vi "Process_Comp_Data.vi"(6 "Queues":T14, 7 "One Seconds in":T11 {"Slave"."Ch1 High" format="%0.0f"; "Master"."Ch1 High" format="%0.0f"}, 8 "Status/Errors in":refnum<vi>, 9 "Get all messages?":bool=TRUE, 10 "Process data parameters out":T1={"Stop loop"={"Settings changed?"=FALSE, "Stop?"=refnum}, "Button refs"={"Stop program"=refnum, "Save settings"=refnum, "DAQ mode"=refnum, "Reset settings"=refnum, "Apply settings"=refnum, "Reset MAS"=refnum, "Reset SLV"=refnum, "Local DBase?"=refnum, "Last value DBase"=FALSE, "Database"=refnum, "Calibration"=refnum, "Save settings 2"=refnum}, "Process messages"={"Process message mode"=enum."Error", "Slave data?"=FALSE, "Length get settings message"=0, "Delta time"=0.0, "Data_Filter"={"Filter_Data"=FALSE, "Use_Thresh"=FALSE, "Reduce data?"=FALSE}, "Time_difference_stack"=[], "Starting sec"=0, "Ending sec"=0, "Ending sec 2"=0, "MAS_Page_Thresh"=refnum, "SLV_Page_Thresh"=refnum, "Database"=refnum}, "Settings state"={"MAS locked?"=refnum, "SLV locked?"=refnum}, "Mode"={"Mode"=enum."Dialog", "Expert?"=FALSE, "Dialog?"=FALSE}, "Alignment parameters"=refnum, "Timer parameters"=refnum, "Files"={"Path config file"=path "", "Path def. ini file"=path "", "Path ini file 1"=path "", "Path ini file 2"=path "", "Path RBF file"=path ""}, "Time difference"=refnum, "Alignment"={"GEN_Page_Calibrate"=refnum, "MAS_Page_Gain"=refnum, "MAS_Page_Offset"=refnum, "SLV_Page_Gain"=refnum, "SLV_Page_Offset"=refnum, "MAS_Page_Common"=refnum, "SLV_Page_Common"=refnum}, "Page Statistics"=refnum}, 11 "Devices in":T10) -> (0 "Status/Errors out":refnum<vi>, 3 "Devices out":T10)   [LabVIEW 2010]
uses:
  Controls/Devices.ctl
  Controls/Queues.ctl
  Controls/One_Second.ctl
  Controls/GPS_Timestamp.ctl
  Controls/One_Seconds.ctl
  Controls/Process_Data_Parameters.ctl
  Controls/Stop_Loop.ctl
  Controls/Button_Refs.ctl
  Controls/Process_Messages.ctl
  Controls/Process_Message_Mode.ctl
  Controls/Settings_State.ctl
  Controls/Mode.ctl
  Controls/Files.ctl
  Controls/Page_Calibration.ctl
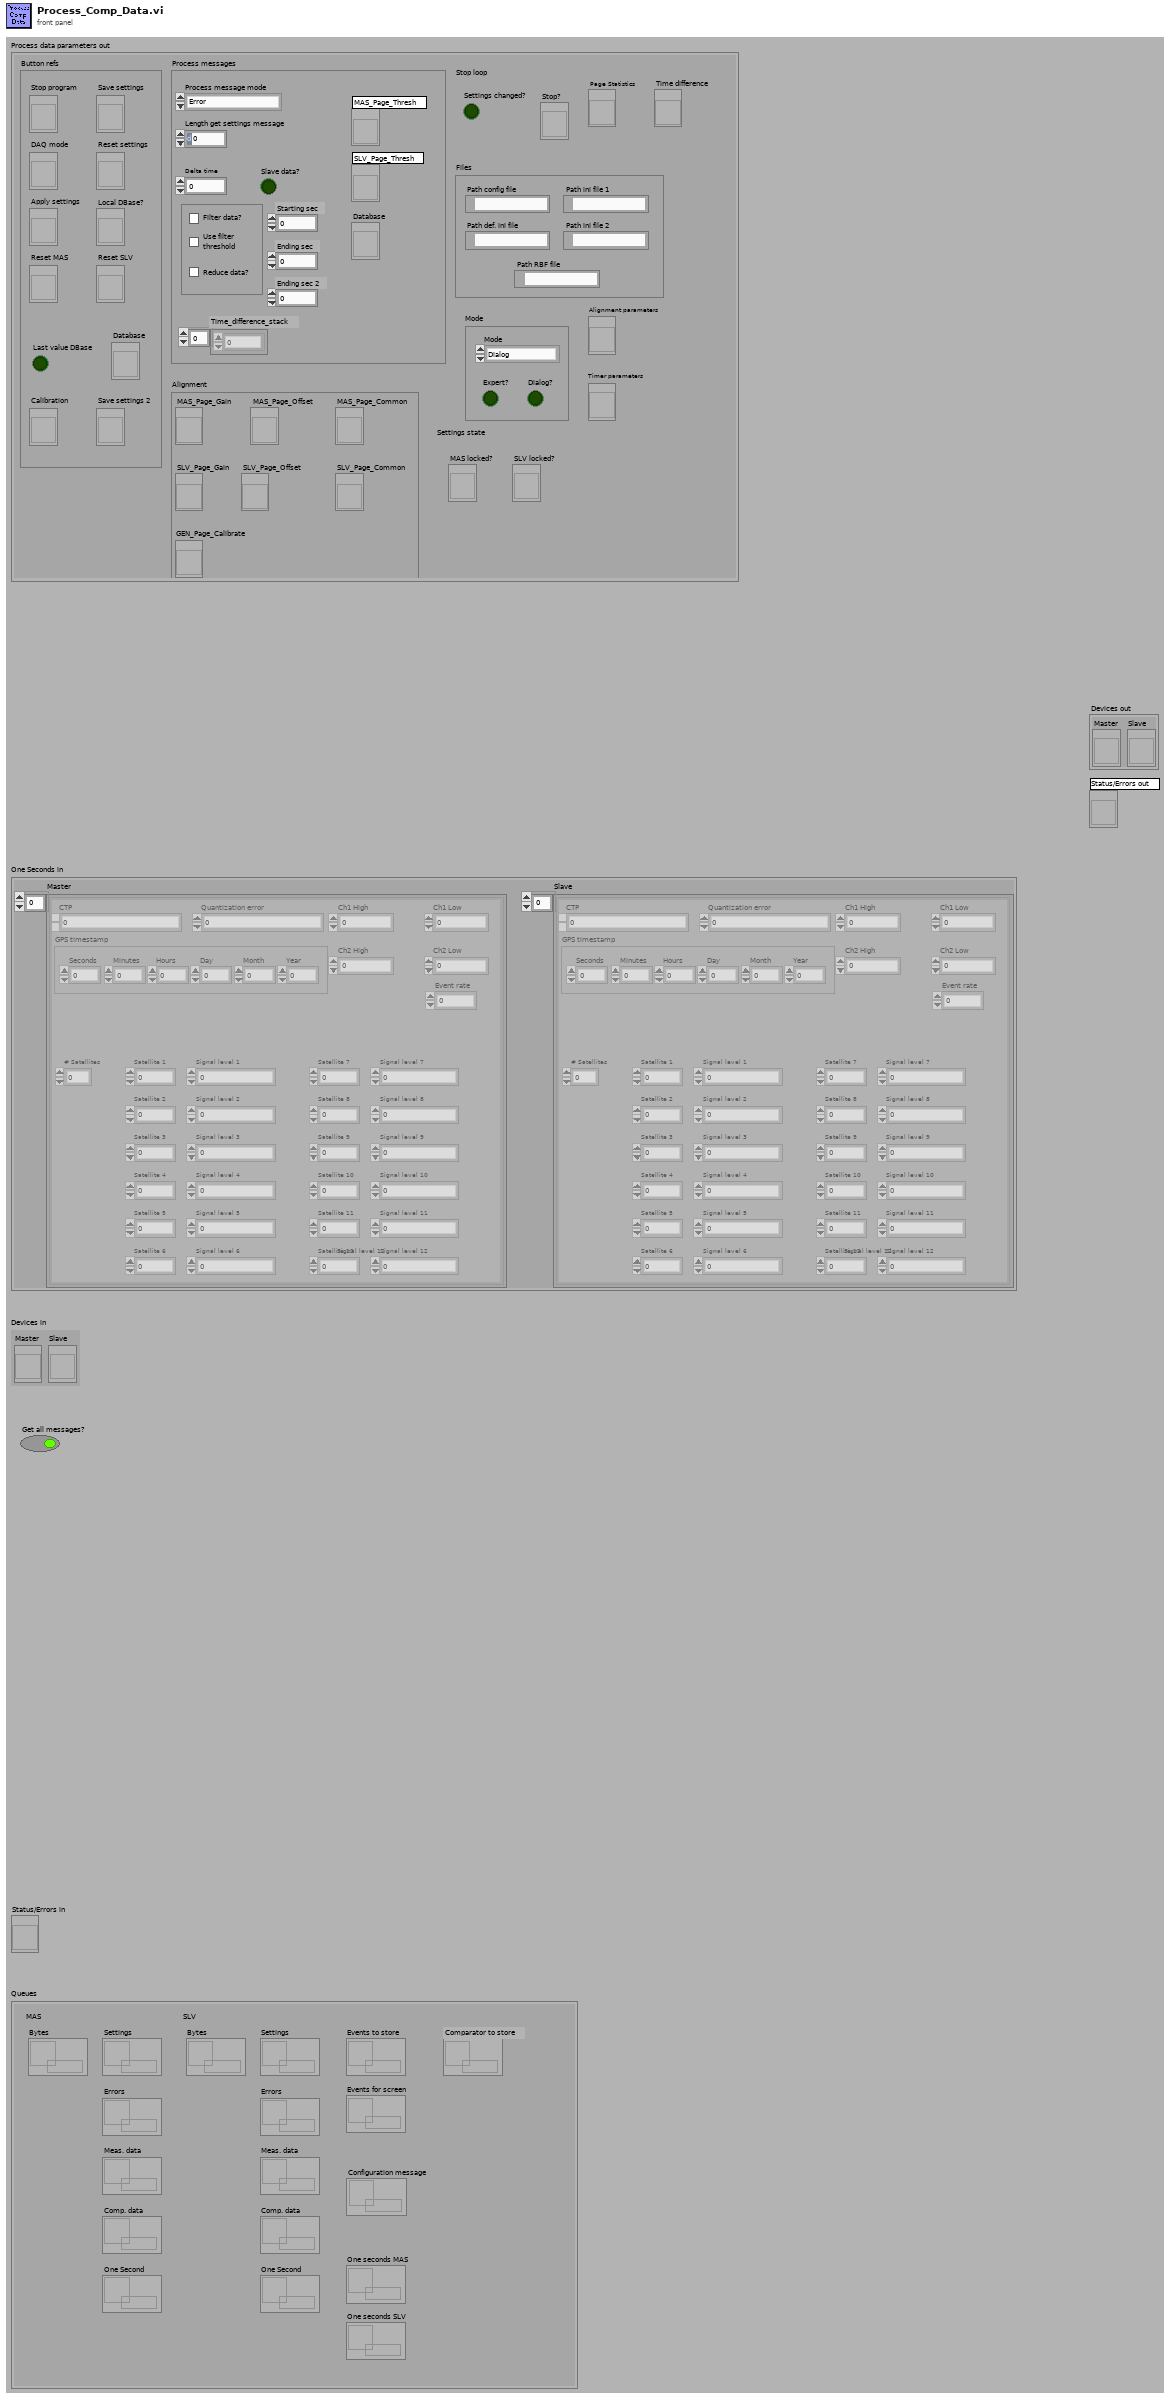
[diagram p1: front panel]
types:
  T1 = typedef "Process_Data_Parameters.ctl" = cluster{"Stop loop":T2, "Button refs":T3, "Process messages":T4, "Settings state":T6, "Mode":T7, "Alignment parameters":refnum<vi>, "Timer parameters":refnum<vi>, "Files":T8, "Time difference":refnum<vi>, "Alignment":T9, "Page Statistics":refnum<vi>}
  T2 = typedef "Stop_Loop.ctl" = cluster{"Settings changed?":bool, "Stop?":refnum<vi>}
  T3 = typedef "Button_Refs.ctl" = cluster{"Stop program":refnum<vi>, "Save settings":refnum<vi>, "DAQ mode":refnum<vi>, "Reset settings":refnum<vi>, "Apply settings":refnum<vi>, "Reset MAS":refnum<vi>, "Reset SLV":refnum<vi>, "Local DBase?":refnum<vi>, "Last value DBase":bool, "Database":refnum<vi>, "Calibration":refnum<vi>, "Save settings 2":refnum<vi>}
  T4 = typedef "Process_Messages.ctl" = cluster{"Process message mode":T5, "Slave data?":bool, "Length get settings message":i32, "Delta time":dbl, "Data_Filter":cluster{"Filter_Data":bool, "Use_Thresh":bool, "Reduce data?":bool}, "Time_difference_stack":u64[], "Starting sec":u64, "Ending sec":u64, "Ending sec 2":u64, "MAS_Page_Thresh":refnum<vi>, "SLV_Page_Thresh":refnum<vi>, "Database":refnum<vi>}
  T5 = typedef "Process_Message_Mode.ctl" = enum16{"Error", "Measurement data", "Comparator data", "One Second"}
  T6 = typedef "Settings_State.ctl" = cluster{"MAS locked?":refnum<vi>, "SLV locked?":refnum<vi>}
  T7 = typedef "Mode.ctl" = cluster{"Mode":enum8{"Stop", "Dialog", "Hisparc II", "Hisparc II DAQ", "Alignment"}, "Expert?":bool, "Dialog?":bool}
  T8 = typedef "Files.ctl" = cluster{"Path config file":path, "Path def. ini file":path, "Path ini file 1":path, "Path ini file 2":path, "Path RBF file":path}
  T9 = typedef "Page_Calibration.ctl" = cluster{"GEN_Page_Calibrate":refnum<vi>, "MAS_Page_Gain":refnum<vi>, "MAS_Page_Offset":refnum<vi>, "SLV_Page_Gain":refnum<vi>, "SLV_Page_Offset":refnum<vi>, "MAS_Page_Common":refnum<vi>, "SLV_Page_Common":refnum<vi>}
  T10 = typedef "Devices.ctl" = cluster{"Master":refnum<vi>, "Slave":refnum<vi>}
  T11 = typedef "One_Seconds.ctl" = cluster{"Master":T12[], "Slave":T12[]}
  T12 = typedef "One_Second.ctl" = cluster{"GPS timestamp":T13, "CTP":u32, "Quantization error":u32, "Ch1 High":u16, "Ch1 Low":u16, "Ch2 High":u16, "Ch2 Low":u16, "Event rate":u16, "# Satellites":u8, "Satellite 1":u8, "Satellite 2":u8, "Satellite 3":u8, "Satellite 4":u8, "Satellite 5":u8, "Satellite 6":u8, "Signal level 1":sgl, "Signal level 2":sgl, "Signal level 3":sgl, "Signal level 4":sgl, "Signal level 5":sgl, "Signal level 6":sgl, "Satellite 7":u8, "Satellite 8":u8, "Satellite 9":u8, "Satellite 10":u8, "Satellite 11":u8, "Satellite 12":u8, "Signal level 7":sgl, "Signal level 8":sgl, "Signal level 9":sgl, "Signal level 10":sgl, "Signal level 11":sgl, "Signal level 12":sgl}
  T13 = typedef "GPS_Timestamp.ctl" = cluster{"Seconds":u8, "Minutes":u8, "Hours":u8, "Day":u8, "Month":u8, "Year":u16}
  T14 = typedef "Queues.ctl" = cluster{"MAS":cluster{"Bytes":refnum<queue>, "Settings":refnum<queue>, "Errors":refnum<queue>, "Meas. data":refnum<queue>, "One Second":refnum<queue>, "Comp. data":refnum<queue>}, "SLV":cluster{"Bytes":refnum<queue>, "Settings":refnum<queue>, "Errors":refnum<queue>, "Meas. data":refnum<queue>, "One Second":refnum<queue>, "Comp. data":refnum<queue>}, "Events to store":refnum<queue>, "Events for screen":refnum<queue>, "One seconds MAS":refnum<queue>, "One seconds SLV":refnum<queue>, "Configuration message":refnum<queue>, "Comparator to store":refnum<queue>}
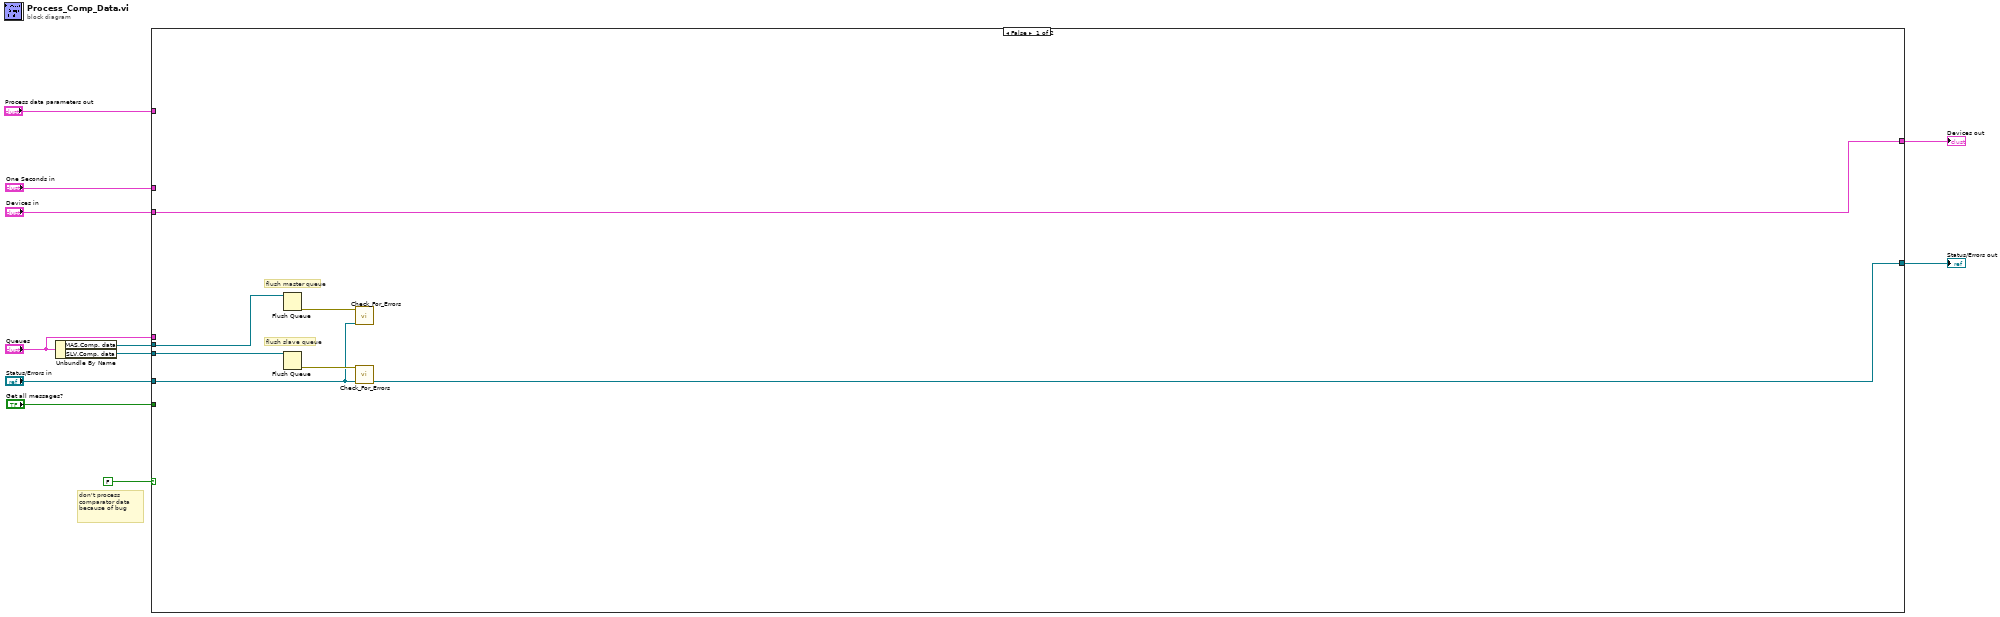
[diagram p0: block diagram]
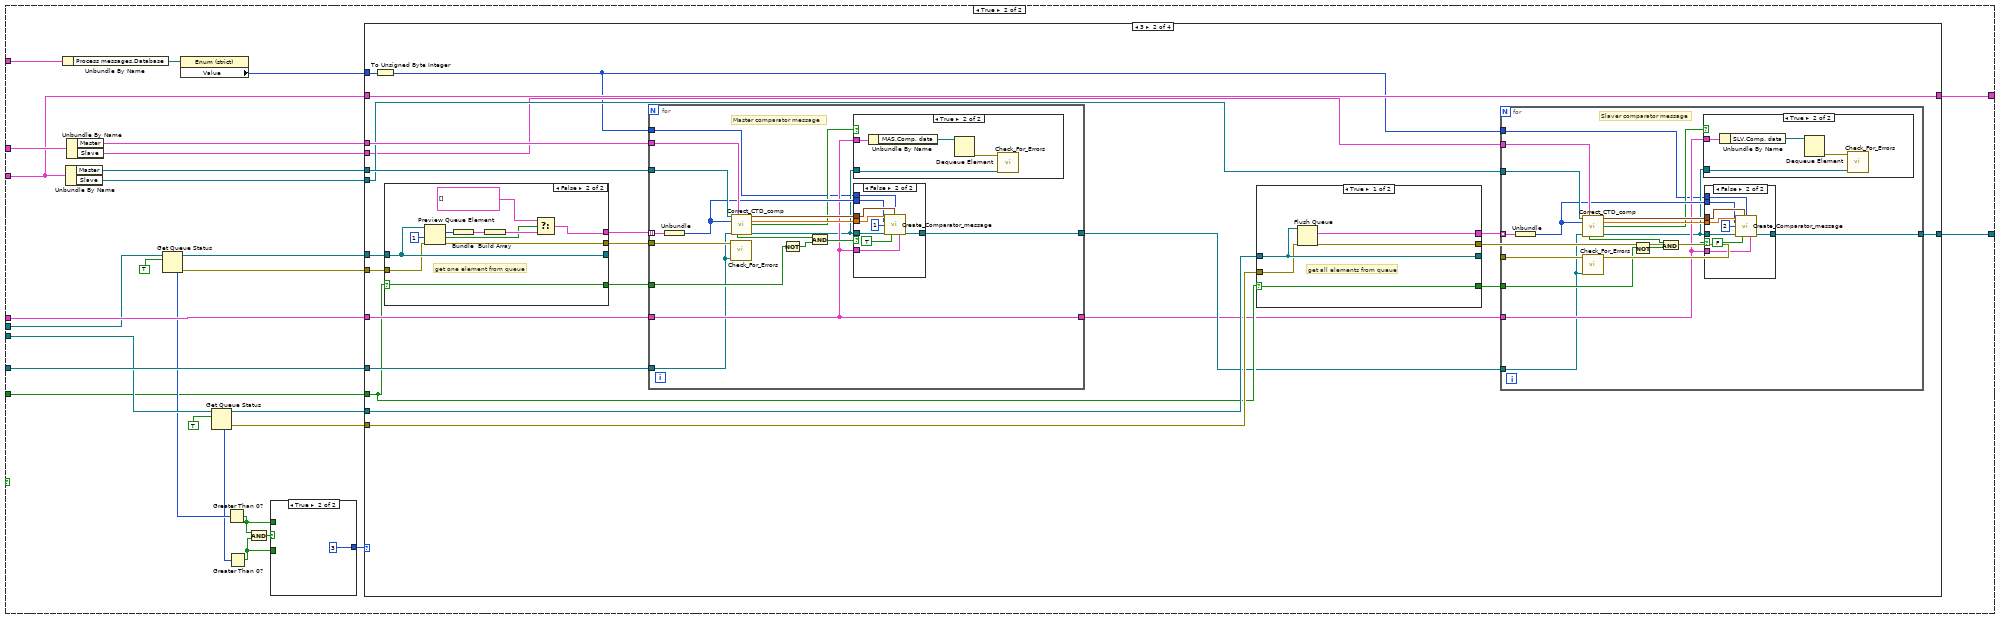
[diagram p2: hidden frame]
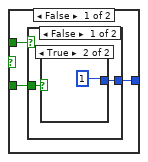
[diagram p3: hidden frame]
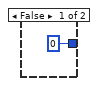
[diagram p4: hidden frame]
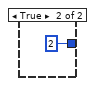
[diagram p5: hidden frame]
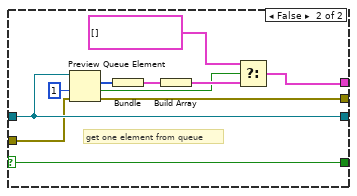
[diagram p7: hidden frame]
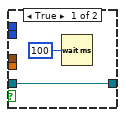
[diagram p9: hidden frame]
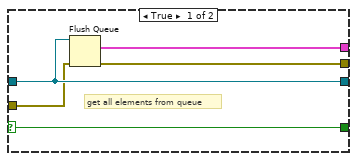
[diagram p10: hidden frame]
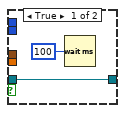
[diagram p12: hidden frame]
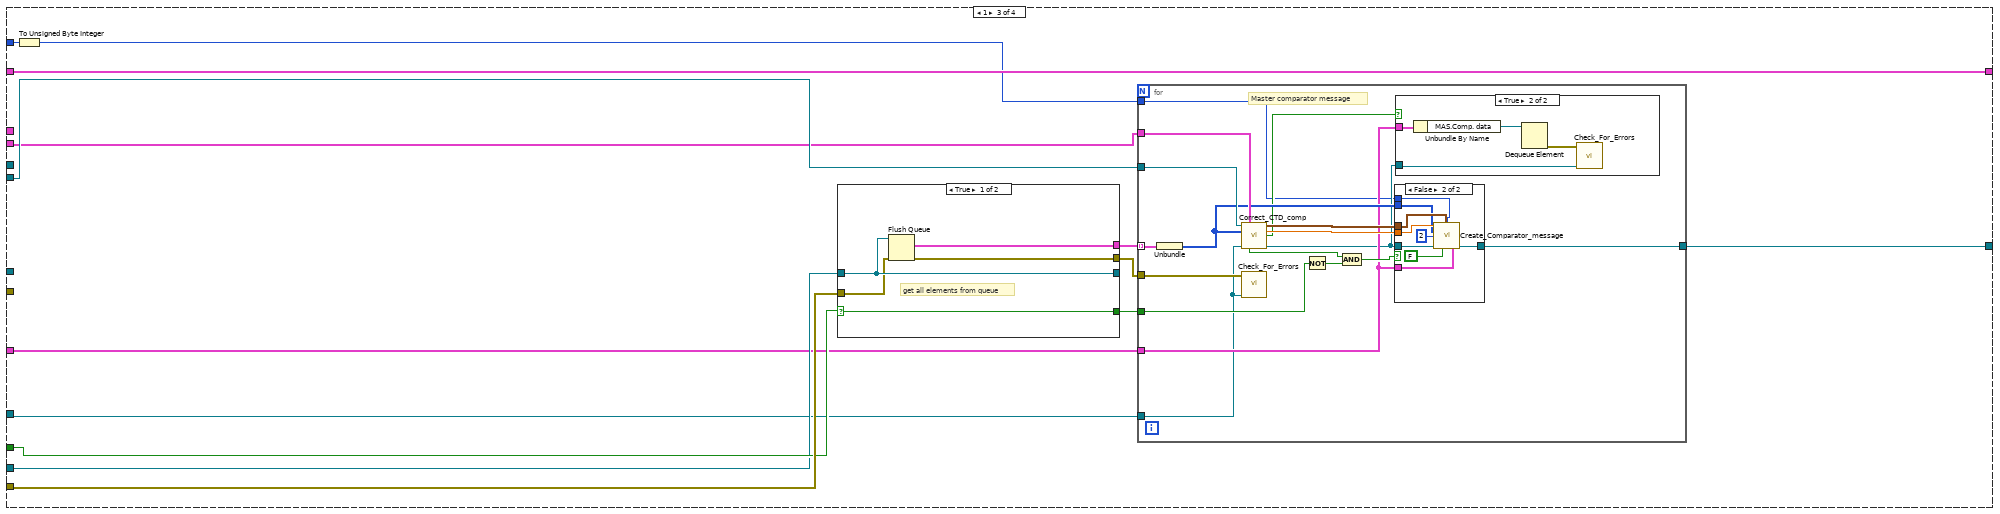
[diagram p13: hidden frame]
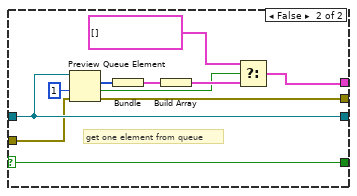
[diagram p14: hidden frame]
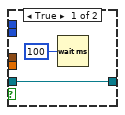
[diagram p16: hidden frame]
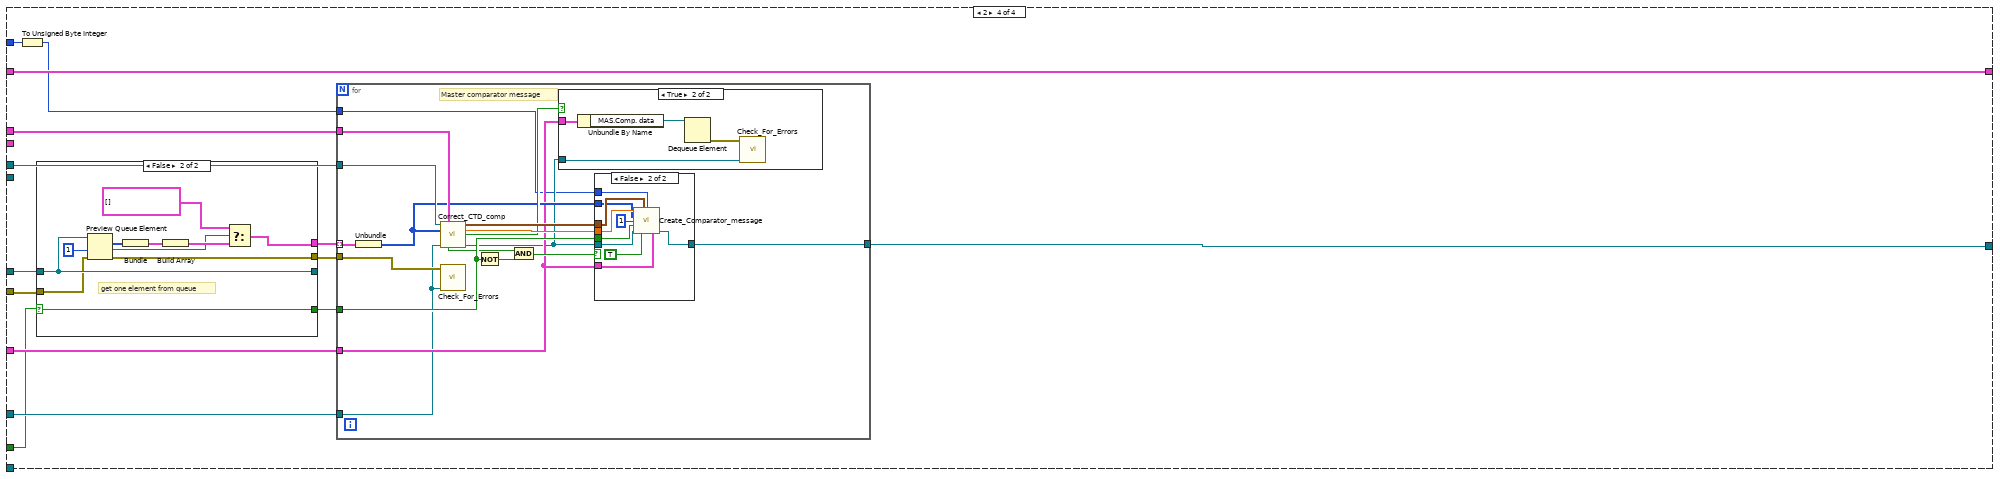
[diagram p17: hidden frame]
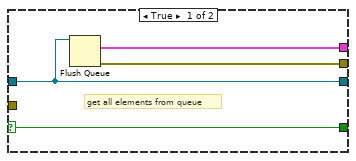
[diagram p18: hidden frame]
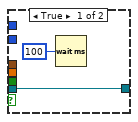
[diagram p20: hidden frame]
diagram:
  # "don't process\ncomparator data\nbecause of bug"
  n1 = Unbundle By Name("Queues") -> ("MAS.Comp. data"=w7:refnum<queue>, "SLV.Comp. data"=w6:refnum<queue>)
  n2 = case shown="False" FALSE {
    tunnel: "One Seconds in" -> [_ w46]
    tunnel: "Status/Errors in" -> [w13 w43]
    tunnel: "Queues" -> [_ w42]
    tunnel: "Devices in" -> [w18 w41]
    tunnel: w7 -> [w17 w34]
    tunnel: w6 -> [w16 w32]
    tunnel: [w18 w24] -> w5
    tunnel: [w12 w23] -> w4
    tunnel: "Get all messages?" -> [_ w22]
    tunnel: "Process data parameters out" -> [_ w21]
    frame False {
      # "flush slave queue"
      # "flush master queue"
      n3 = Flush Queue(queue=w17) -> (error out=w15:errorcluster)  [unwired: 1 in, 2 out]
      n4 = Flush Queue(queue=w16) -> (error out=w14:errorcluster)  [unwired: 1 in, 2 out]
      n5 = call "Check_For_Errors.vi"("Status/Errors in"=w13, "error in"=w15) -> ()  [unwired: 10 out]
      n6 = call "Check_For_Errors.vi"("Status/Errors in"=w13, "error in"=w14) -> ("Status/Errors out"=w12:refnum<vi>)  [unwired: 9 out]
    }
    frame True {
      n7 = Unbundle By Name(w21) -> ("Process messages.Database"=w20:refnum<vi>)
      n8 = Unbundle By Name(w41) -> ("Master"=w39:refnum<vi>, "Slave"=w44:refnum<vi>)
      n9 = Unbundle By Name(w46) -> ("Master"=w45:T12[], "Slave"=w40:T12[])
      n10 = Get Queue Status(queue=w34, return elements? (F)=TRUE) -> (queue out=w35:refnum<queue>, error out=w25:errorcluster, # elements in queue=w29:i32)  [unwired: 1 in, 5 out]
      n11 = property class="Enum (strict)"(reference=w20) -> ("Value"=w19:enum8{"none", "local", "central", "both"})  [unwired: 1 in, 2 out]
      n12 = Get Queue Status(queue=w32, return elements? (F)=TRUE) -> (queue out=w33:refnum<queue>, error out=w26:errorcluster, # elements in queue=w28:i32)  [unwired: 1 in, 5 out]
      n13 = Greater Than 0?(x=w29) -> (x > 0?=w37:bool)
      n14 = Greater Than 0?(x=w28) -> (x > 0?=w36:bool)
      n15 = And(x=w37, y=w36) -> (x .and. y?=w38:bool)
      n16 = case shown="True" w38 {
        tunnel: [w48 3] -> w27
        tunnel: w37 -> [w49 _]
        tunnel: w36 -> [w47 _]
        frame False {
          n17 = case shown="False" w49 {
            tunnel: [w50 2] -> w48
            tunnel: w47 -> [w51 _]
            frame False {
              n18 = case shown="True" w51 {
                tunnel: [0 1] -> w50
                frame False {
                }
                frame True {
                }
              }
            }
            frame True {
            }
          }
        }
        frame True {
        }
      }
      n19 = case shown="3" w27 {
        tunnel: w45 -> [_ w73 _ w249]
        tunnel: w44 -> [_ w68 w185 _]
        tunnel: w43 -> [w57 w72 w179 w241]
        tunnel: w42 -> [_ w77 w178 w244]
        tunnel: w35 -> [_ w75 _ w245]
        tunnel: w41 -> [w56 w61 w181 w247]
        tunnel: w40 -> [_ w60 w177 _]
        tunnel: w39 -> [_ w74 _ w248]
        tunnel: w33 -> [_ w67 w180 _]
        tunnel: w26 -> [_ w66 w184 _]
        tunnel: w25 -> [_ w76 _ w240]
        tunnel: [w56 w61 w181 w247] -> w24
        tunnel: [w57 w62 w182 w246] -> w23
        tunnel: w22 -> [_ w65 w183 w239]
        tunnel: w19 -> [_ w59 w176 w237]
        frame 0, Default {
        }
        frame 3 {
          n20 = To Unsigned Byte Integer(number=w59) -> (unsigned 8bit integer=w58:u8)
          n21 = case shown="False" w65 {
            selector: w65 -> [w129 w133]
            tunnel: [w132 w143] -> w79
            tunnel: w75 -> [w130 w140]
            tunnel: [w131 w136] -> w80
            tunnel: [w130 w140] -> _
            tunnel: w76 -> [w128 w134]
            tunnel: [w129 w133] -> w78
            frame True {
              # "get all elements from queue"
              n22 = Flush Queue(queue=w130, error in (no error)=w128) -> (remaining elements=w131:cluster{u8[]}[], error out=w132:errorcluster)  [unwired: 1 out]
            }
            frame False {
              # "get one element from queue"
              n23 = Preview Queue Element(queue=w140, timeout in ms (-1)=1, error in (no error)=w134) -> (element=w142:u8[], timed out?=w137:bool, error out=w143:errorcluster)  [unwired: 1 out]
              n24 = Bundle(w142) -> (w141:cluster{u8[]})  [unwired: 1 in]
              n25 = Build Array(w141) -> (w138:cluster{u8[]}[])
              n26 = Select(t=cluster{u8[]}[] [], s=w137, f=w138) -> (s? t:f=w136:cluster{u8[]}[])
            }
          }
          n27 = for {
            tunnel: w74 -> [w154]
            tunnel: w79 -> [w159]
            tunnel: w77 -> [w147]
            tunnel: w80 -> [w155] mode=indexing
            tunnel: [w156] -> w64
            tunnel: w72 -> [w145]
            tunnel: w78 -> [w149]
            tunnel: [w147] -> w63
            tunnel: w73 -> [w153]
            tunnel: w58 -> [w144]
            # "Master comparator message"
            n28 = Unbundle(w155) -> (w148:u8[])
            n29 = call "Check_For_Errors.vi"("Status/Errors in"=w145, "error in"=w159) -> ()  [unwired: 10 out]
            n30 = call "Correct_CTD_comp.vi"("Device in"=w154, "One Second in"=w153, "Message in"=w148, "Status/Errors in"=w145) -> ("GPS timestamp out"=w157:T13, "Time"=w158:dbl, "No 1 sec?"=w146:bool, "Wait for tick count?"=w150:bool)  [unwired: 8 out]
            n31 = Not(x=w149) -> (.not. x?=w152:bool)
            n32 = And(x=w150, y=w152) -> (x .and. y?=w151:bool)
            n33 = case shown="True" w146 {
              tunnel: w147 -> [_ w163]
              tunnel: w145 -> [_ w160]
              frame False {
              }
              frame True {
                n34 = Unbundle By Name(w163) -> ("MAS.Comp. data"=w162:refnum<queue>)
                n35 = Dequeue Element(queue=w162) -> (error out=w161:errorcluster)  [unwired: 1 in, 4 out]
                n36 = call "Check_For_Errors.vi"("Status/Errors in"=w160, "error in"=w161) -> ()  [unwired: 10 out]
              }
            }
            n37 = case shown="False" w151 {
              tunnel: w147 -> [_ w173]
              tunnel: w158 -> [_ w172]
              tunnel: w157 -> [_ w171]
              tunnel: [w165 w170] -> w156
              tunnel: w148 -> [_ w169]
              tunnel: w145 -> [w165 w168]
              tunnel: w144 -> [_ w166]
              frame True {
                n38 = Wait (ms)(milliseconds to wait=u32 100) -> ()  [unwired: 1 out]
              }
              frame False {
                n39 = call "Create_Comparator_message.vi"("Time"=w172, "GPS timestamp"=w171, "Database"=w166, "Array"=w169, "Device identifier"=u8 1, "Status/Errors in"=w168, "Master?"=TRUE, "Queues"=w173) -> ("Status/Errors out"=w170:refnum<vi>)  [unwired: 2 in, 5 out]
              }
            }
          }
          n40 = case shown="True" w65 {
            selector: w65 -> [w82 w86]
            tunnel: [w85 w96] -> w70
            tunnel: w67 -> [w83 w93]
            tunnel: [w84 w89] -> w71
            tunnel: [w83 w93] -> _
            tunnel: w66 -> [w81 w87]
            tunnel: [w82 w86] -> w69
            frame True {
              # "get all elements from queue"
              n41 = Flush Queue(queue=w83, error in (no error)=w81) -> (remaining elements=w84:cluster{u8[]}[], error out=w85:errorcluster)  [unwired: 1 out]
            }
            frame False {
              # "get one element from queue"
              n42 = Preview Queue Element(queue=w93, timeout in ms (-1)=1, error in (no error)=w87) -> (element=w95:u8[], timed out?=w90:bool, error out=w96:errorcluster)  [unwired: 1 out]
              n43 = Bundle(w95) -> (w94:cluster{u8[]})  [unwired: 1 in]
              n44 = Build Array(w94) -> (w91:cluster{u8[]}[])
              n45 = Select(t=cluster{u8[]}[] [], s=w90, f=w91) -> (s? t:f=w89:cluster{u8[]}[])
            }
          }
          n46 = for {
            tunnel: w68 -> [w107]
            tunnel: w70 -> [w112]
            tunnel: w63 -> [w100]
            tunnel: w71 -> [w108] mode=indexing
            tunnel: [w109] -> w62
            tunnel: w64 -> [w99]
            tunnel: w69 -> [w102]
            tunnel: w60 -> [w106]
            tunnel: w58 -> [w97]
            # "Slaver comparator message"
            n47 = Unbundle(w108) -> (w101:u8[])
            n48 = call "Correct_CTD_comp.vi"("Device in"=w107, "One Second in"=w106, "Message in"=w101, "Status/Errors in"=w99) -> ("GPS timestamp out"=w110:T13, "Time"=w111:dbl, "No 1 sec?"=w98:bool, "Wait for tick count?"=w103:bool)  [unwired: 8 out]
            n49 = call "Check_For_Errors.vi"("Status/Errors in"=w99, "error in"=w112) -> ()  [unwired: 10 out]
            n50 = Not(x=w102) -> (.not. x?=w105:bool)
            n51 = And(x=w103, y=w105) -> (x .and. y?=w104:bool)
            n52 = case shown="True" w98 {
              tunnel: w100 -> [_ w116]
              tunnel: w99 -> [_ w113]
              frame False {
              }
              frame True {
                n53 = Unbundle By Name(w116) -> ("SLV.Comp. data"=w115:refnum<queue>)
                n54 = Dequeue Element(queue=w115) -> (error out=w114:errorcluster)  [unwired: 1 in, 4 out]
                n55 = call "Check_For_Errors.vi"("Status/Errors in"=w113, "error in"=w114) -> ()  [unwired: 10 out]
              }
            }
            n56 = case shown="False" w104 {
              tunnel: w100 -> [_ w126]
              tunnel: w111 -> [_ w125]
              tunnel: w110 -> [_ w124]
              tunnel: [w118 w123] -> w109
              tunnel: w101 -> [_ w122]
              tunnel: w99 -> [w118 w121]
              tunnel: w97 -> [_ w119]
              frame True {
                n57 = Wait (ms)(milliseconds to wait=u32 100) -> ()  [unwired: 1 out]
              }
              frame False {
                n58 = call "Create_Comparator_message.vi"("Time"=w125, "GPS timestamp"=w124, "Database"=w119, "Array"=w122, "Device identifier"=u8 2, "Status/Errors in"=w121, "Master?"=FALSE, "Queues"=w126) -> ("Status/Errors out"=w123:refnum<vi>)  [unwired: 2 in, 5 out]
              }
            }
          }
        }
        frame 1 {
          n59 = To Unsigned Byte Integer(number=w176) -> (unsigned 8bit integer=w175:u8)
          n60 = case shown="True" w183 {
            selector: w183 -> [w190 w194]
            tunnel: [w193 w204] -> w187
            tunnel: w180 -> [w191 w201]
            tunnel: [w192 w197] -> w188
            tunnel: [w191 w201] -> _
            tunnel: w184 -> [w189 w195]
            tunnel: [w190 w194] -> w186
            frame True {
              # "get all elements from queue"
              n61 = Flush Queue(queue=w191, error in (no error)=w189) -> (remaining elements=w192:cluster{u8[]}[], error out=w193:errorcluster)  [unwired: 1 out]
            }
            frame False {
              # "get one element from queue"
              n62 = Preview Queue Element(queue=w201, timeout in ms (-1)=1, error in (no error)=w195) -> (element=w203:u8[], timed out?=w198:bool, error out=w204:errorcluster)  [unwired: 1 out]
              n63 = Bundle(w203) -> (w202:cluster{u8[]})  [unwired: 1 in]
              n64 = Build Array(w202) -> (w199:cluster{u8[]}[])
              n65 = Select(t=cluster{u8[]}[] [], s=w198, f=w199) -> (s? t:f=w197:cluster{u8[]}[])
            }
          }
          n66 = for {
            tunnel: w185 -> [w215]
            tunnel: w187 -> [w220]
            tunnel: w178 -> [w208]
            tunnel: w188 -> [w216] mode=indexing
            tunnel: [w217] -> w182
            tunnel: w179 -> [w207]
            tunnel: w186 -> [w210]
            tunnel: w177 -> [w214]
            tunnel: w175 -> [w205]
            # "Master comparator message"
            n67 = Unbundle(w216) -> (w209:u8[])
            n68 = call "Correct_CTD_comp.vi"("Device in"=w215, "One Second in"=w214, "Message in"=w209, "Status/Errors in"=w207) -> ("GPS timestamp out"=w218:T13, "Time"=w219:dbl, "No 1 sec?"=w206:bool, "Wait for tick count?"=w211:bool)  [unwired: 8 out]
            n69 = call "Check_For_Errors.vi"("Status/Errors in"=w207, "error in"=w220) -> ()  [unwired: 10 out]
            n70 = Not(x=w210) -> (.not. x?=w213:bool)
            n71 = And(x=w211, y=w213) -> (x .and. y?=w212:bool)
            n72 = case shown="False" w212 {
              tunnel: w208 -> [_ w234]
              tunnel: w219 -> [_ w233]
              tunnel: w218 -> [_ w232]
              tunnel: [w226 w231] -> w217
              tunnel: w209 -> [_ w230]
              tunnel: w207 -> [w226 w229]
              tunnel: w205 -> [_ w227]
              frame True {
                n73 = Wait (ms)(milliseconds to wait=u32 100) -> ()  [unwired: 1 out]
              }
              frame False {
                n74 = call "Create_Comparator_message.vi"("Time"=w233, "GPS timestamp"=w232, "Database"=w227, "Array"=w230, "Device identifier"=u8 2, "Status/Errors in"=w229, "Master?"=FALSE, "Queues"=w234) -> ("Status/Errors out"=w231:refnum<vi>)  [unwired: 2 in, 5 out]
              }
            }
            n75 = case shown="True" w206 {
              tunnel: w208 -> [_ w224]
              tunnel: w207 -> [_ w221]
              frame False {
              }
              frame True {
                n76 = Unbundle By Name(w224) -> ("MAS.Comp. data"=w223:refnum<queue>)
                n77 = Dequeue Element(queue=w223) -> (error out=w222:errorcluster)  [unwired: 1 in, 4 out]
                n78 = call "Check_For_Errors.vi"("Status/Errors in"=w221, "error in"=w222) -> ()  [unwired: 10 out]
              }
            }
          }
        }
        frame 2 {
          n79 = To Unsigned Byte Integer(number=w237) -> (unsigned 8bit integer=w236:u8)
          n80 = case shown="False" w239 {
            selector: w239 -> [w250 w254]
            tunnel: [w253 w264] -> w242
            tunnel: w245 -> [w251 w261]
            tunnel: [w252 w257] -> w243
            tunnel: [w251 w261] -> _
            tunnel: w240 -> [_ w255]
            tunnel: [w250 w254] -> w238
            frame True {
              # "get all elements from queue"
              n81 = Flush Queue(queue=w251) -> (remaining elements=w252:cluster{u8[]}[], error out=w253:errorcluster)  [unwired: 1 in, 1 out]
            }
            frame False {
              # "get one element from queue"
              n82 = Preview Queue Element(queue=w261, timeout in ms (-1)=1, error in (no error)=w255) -> (element=w263:u8[], timed out?=w258:bool, error out=w264:errorcluster)  [unwired: 1 out]
              n83 = Bundle(w263) -> (w262:cluster{u8[]})  [unwired: 1 in]
              n84 = Build Array(w262) -> (w259:cluster{u8[]}[])
              n85 = Select(t=cluster{u8[]}[] [], s=w258, f=w259) -> (s? t:f=w257:cluster{u8[]}[])
            }
          }
          n86 = for {
            tunnel: w248 -> [w275]
            tunnel: w242 -> [w280]
            tunnel: w244 -> [w267]
            tunnel: w243 -> [w276] mode=indexing
            tunnel: [w277] -> w246
            tunnel: w241 -> [w266]
            tunnel: w238 -> [w272]
            tunnel: w249 -> [w274]
            tunnel: w236 -> [w265]
            # "Master comparator message"
            n87 = Unbundle(w276) -> (w268:u8[])
            n88 = call "Correct_CTD_comp.vi"("Device in"=w275, "One Second in"=w274, "Message in"=w268, "Status/Errors in"=w266) -> ("GPS timestamp out"=w278:T13, "Time"=w279:dbl, "No 1 sec?"=w269:bool, "Wait for tick count?"=w271:bool)  [unwired: 8 out]
            n89 = call "Check_For_Errors.vi"("Status/Errors in"=w266, "error in"=w280) -> ()  [unwired: 10 out]
            n90 = Not(x=w272) -> (.not. x?=w273:bool)
            n91 = And(x=w271, y=w273) -> (x .and. y?=w270:bool)
            n92 = case shown="True" w269 {
              tunnel: w267 -> [_ w284]
              tunnel: w266 -> [_ w281]
              frame False {
              }
              frame True {
                n93 = Unbundle By Name(w284) -> ("MAS.Comp. data"=w283:refnum<queue>)
                n94 = Dequeue Element(queue=w283) -> (error out=w282:errorcluster)  [unwired: 1 in, 4 out]
                n95 = call "Check_For_Errors.vi"("Status/Errors in"=w281, "error in"=w282) -> ()  [unwired: 10 out]
              }
            }
            n96 = case shown="False" w270 {
              tunnel: w267 -> [_ w295]
              tunnel: w279 -> [_ w294]
              tunnel: w278 -> [_ w293]
              tunnel: [w286 w292] -> w277
              tunnel: w268 -> [_ w291]
              tunnel: w266 -> [w286 w290]
              tunnel: w272 -> [_ w288]
              tunnel: w265 -> [_ w287]
              frame True {
                n97 = Wait (ms)(milliseconds to wait=u32 100) -> ()  [unwired: 1 out]
              }
              frame False {
                n98 = call "Create_Comparator_message.vi"("Time"=w294, "GPS timestamp"=w293, "Database"=w287, "Array"=w291, "Device identifier"=u8 1, "Get all elements?"=w288, "Status/Errors in"=w290, "Master?"=TRUE, "Queues"=w295) -> ("Status/Errors out"=w292:refnum<vi>)  [unwired: 1 in, 5 out]
              }
            }
          }
        }
      }
    }
  }
  "Devices out" <- w5
  "Status/Errors out" <- w4
